vi "Hysteresis-SimulateHysteresis.vi"(9 "Polynomial Coefficients":dbl[](array[numeric]), 10 "Relative Range":dbl, 11 "NbPoints":i32) -> (3 "Hyst curve":dbl[](array[numeric]))   [LabVIEW 2016]
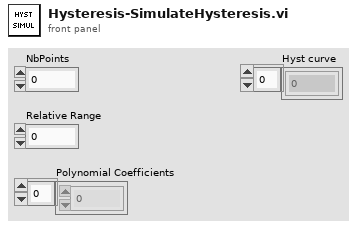
[diagram p1: front panel]
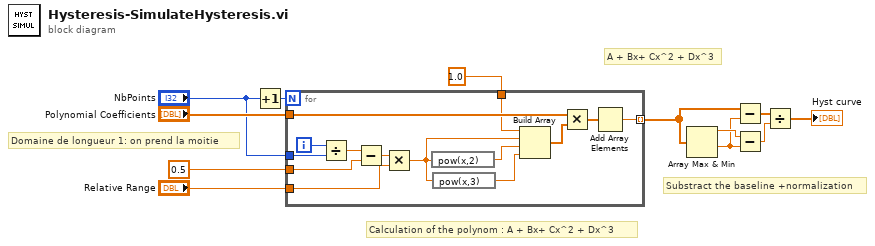
[diagram p0: block diagram]
diagram:
  # "Substract the baseline +normalization"
  # "A + Bx+ Cx^2 + Dx^3"
  # "Calculation of the polynom : A + Bx+ Cx^2 + Dx^3"
  # "Domaine de longueur 1: on prend la moitie"
  n1 = Increment(x="NbPoints") -> (x+1=w1:i32)
  n2 = for {
    N: w1 -> [_]
    tunnel: "NbPoints" -> [w25]
    tunnel: [w22] -> w8 mode=indexing
    tunnel: "Relative Range" -> [w19]
    tunnel: "Polynomial Coefficients" -> [w18]
    tunnel: 0.5 ("y") -> [w16]
    tunnel: 1.0 -> [w13]
    i -> [w26]
    n3 = Divide(x=w26, y=w25) -> (x/y=w20:dbl)
    n4 = Subtract(x=w20, y=w16) -> (x-y=w21:dbl)
    n5 = Multiply(x=w21, y=w19) -> (x*y=w15:dbl)
    n6 = expression code="pow(x,2)"(w15) -> (w14:dbl)
    n7 = expression code="pow(x,3)"(w15) -> (w17:dbl)
    n8 = Build Array(w13, w15, w14, w17) -> (w24:dbl[])
    n9 = Multiply(x=w18, y=w24) -> (x*y=w23:dbl[])
    n10 = Add Array Elements(numeric array=w23) -> (sum=w22:dbl)
  }
  n11 = Array Max & Min(array=w8) -> (max value=w7:dbl, min value=w6:dbl)  [unwired: 2 out]
  n12 = Subtract(x=w8, y=w6) -> (x-y=w5:dbl[])
  n13 = Subtract(x=w7, y=w6) -> (x-y=w4:dbl)
  n14 = Divide(x=w5, y=w4) -> (x/y=→"Hyst curve":dbl[])
